vi "microspec_validating_v9.vi"() -> ()   [LabVIEW 2009]
uses:
  <vilib>/Utility/file.llb/Write To Spreadsheet File (string).vi
  <vilib>/Instr/_visa.llb/VISA Configure Serial Port (Instr).vi
panel:
  in  "Path":path
  in  "intergration time":dbl caption="sensor\nintergration time (us)" min=54.0 max=5000000.0 step=100.0
  in  "?":T1(tab)
  out "radiometer data file path":path
  in  "Runname":string
  out "Sensor_name":string
  out "Radiometer Average":dbl
  in  "Delay":dbl
  in  "Step":dbl
  in  "Stop Wl":dbl min=0.0 max=5000.0 step=100.0
  in  "Start Wl":dbl min=0.0 max=5000.0 step=100.0
  in  "mean_number":i32 caption="Mean Number"
  out "Current Wavelength":dbl
  out "XY-Graph 2":cluster{"Y":dbl[], "Y":dbl[]}[](graph)
  in  "run 5":bool
  out "sectrometer data file path":path
  in  "save data":bool
  in  "reset with every wavelength?":bool caption="reset with new run?"
  in  "Delay":dbl
  in  "Step":dbl
  in  "Stop Wl":dbl min=0.0 max=5000.0 step=100.0
  out "Current Wavelength":dbl
  in  "Start Wl 2":dbl min=0.0 max=5000.0 step=10.0
  in  "Sensor":string(combo)
  in  "run 2":bool
  in  "Set Runs":i32
  out "Current Run":i32
  in  "stop runs":bool
  out "raw_data":cluster{"Y":dbl[], "Y":dbl[]}[](graph) caption="raw data"
  out "raw_data 2":cluster{"Y":dbl[], "Y":dbl[]}[](graph) caption="raw data"
  in  "Stopp":bool
  out "System Setup":i32
  out "DLL Version":string
  out "Get Version":i32
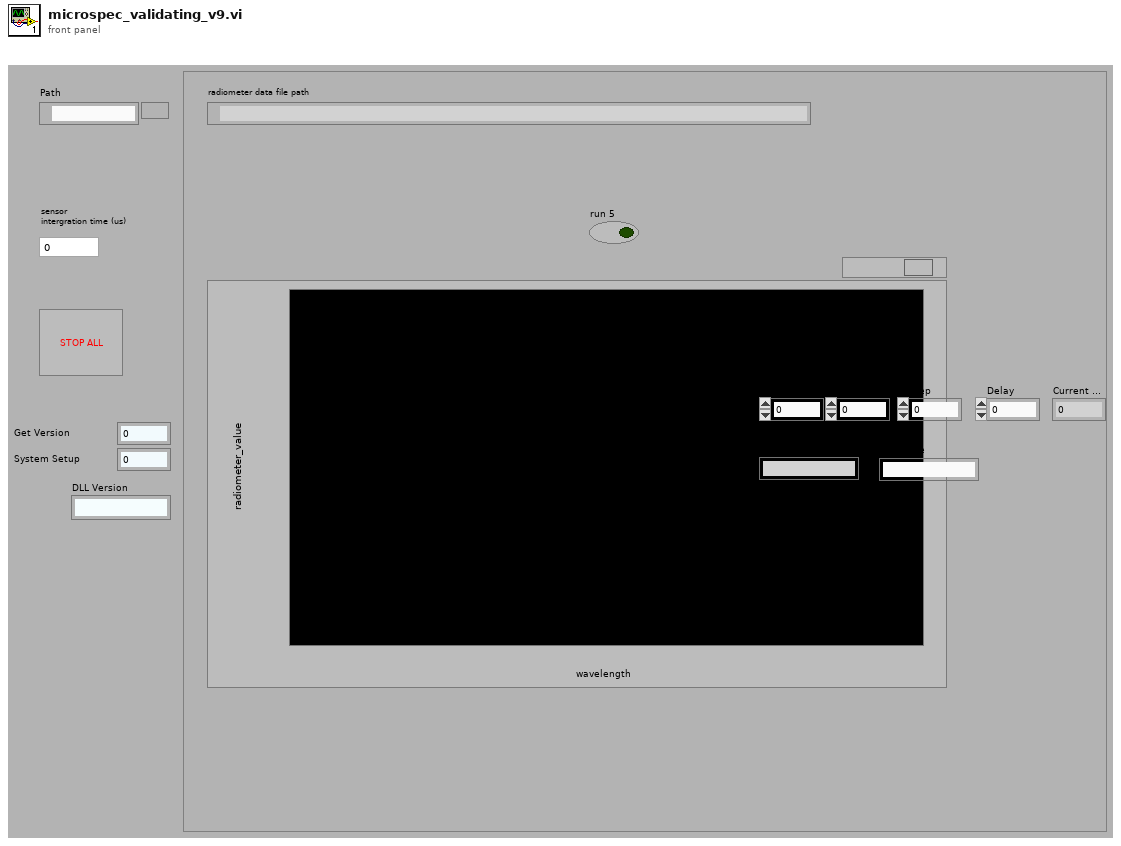
[diagram p1: front panel]
types:
  T1 = enum32{"radiometer calibration", "measuring sequence", "microspec standalone"}
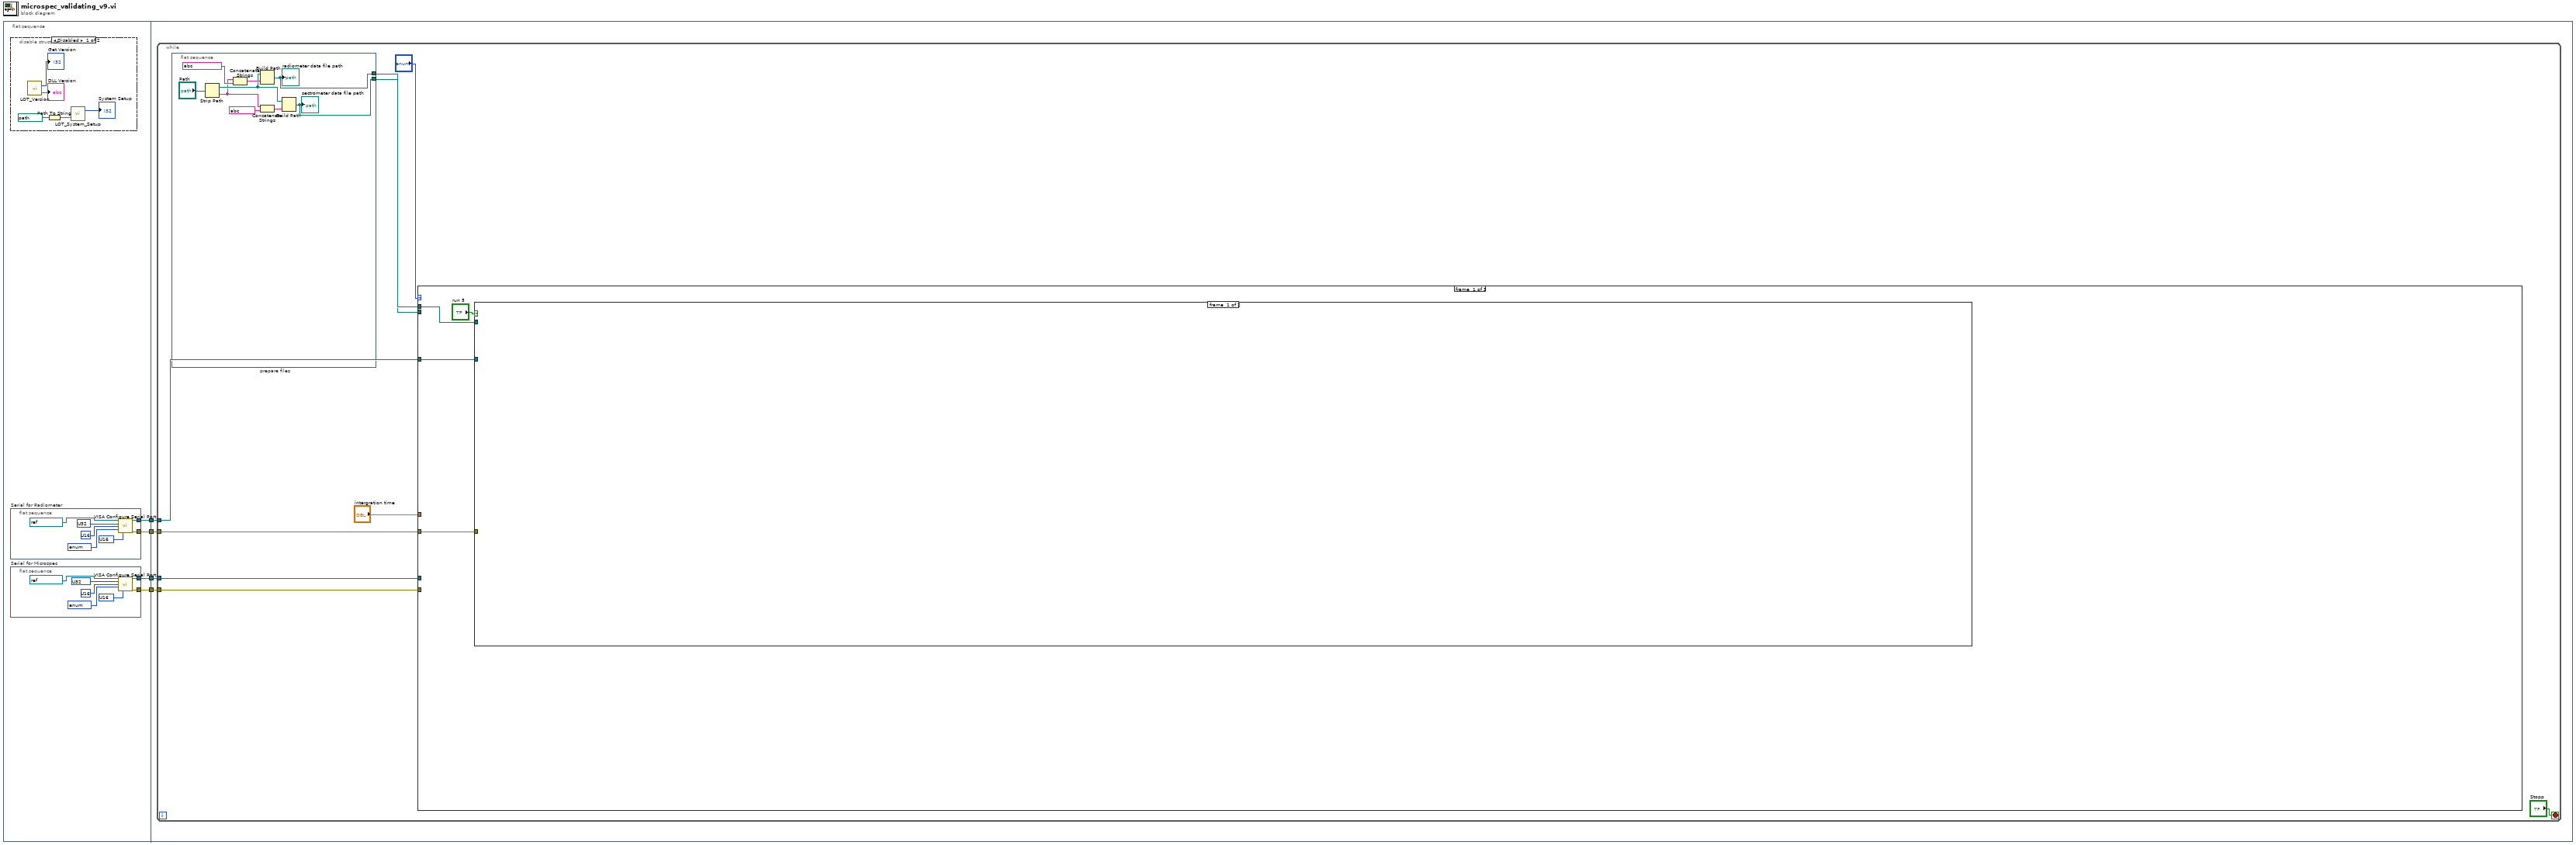
[diagram p0: block diagram]
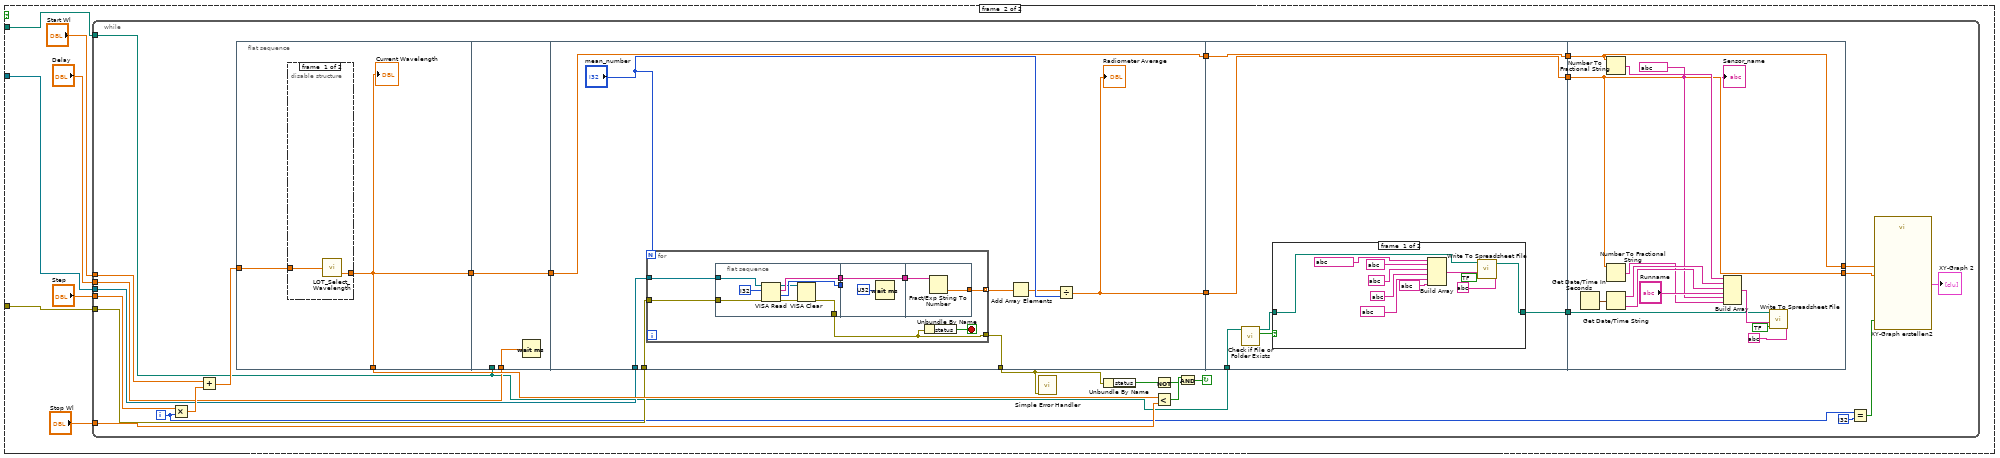
[diagram p3: hidden frame]
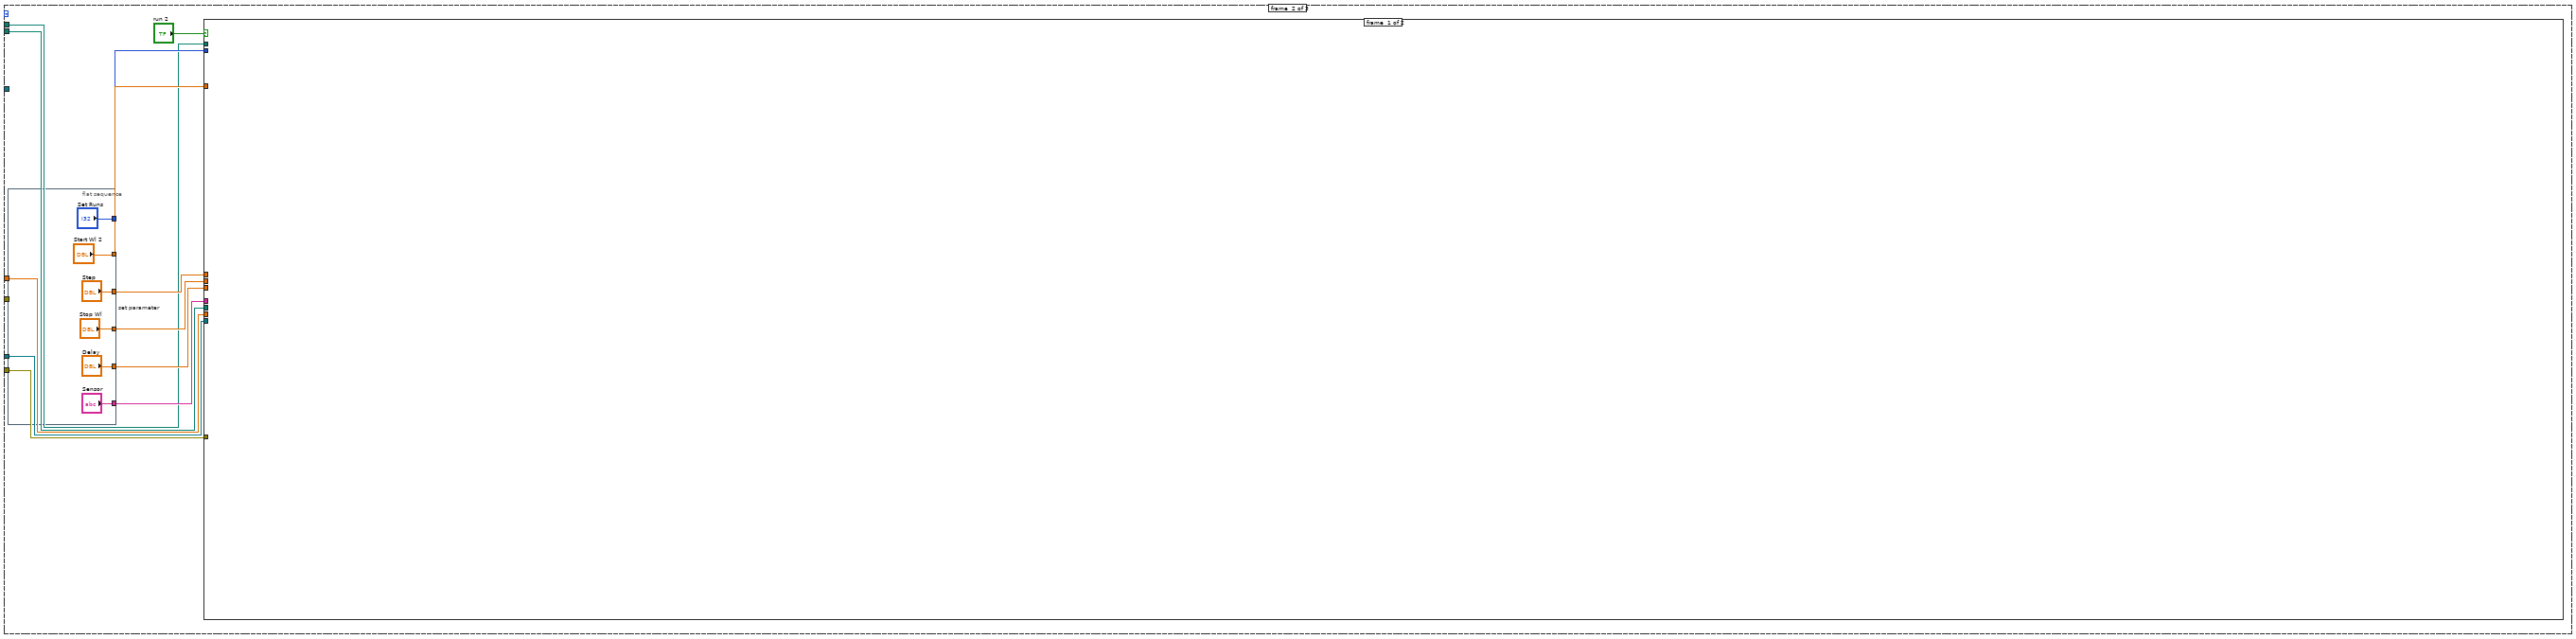
[diagram p6: hidden frame]
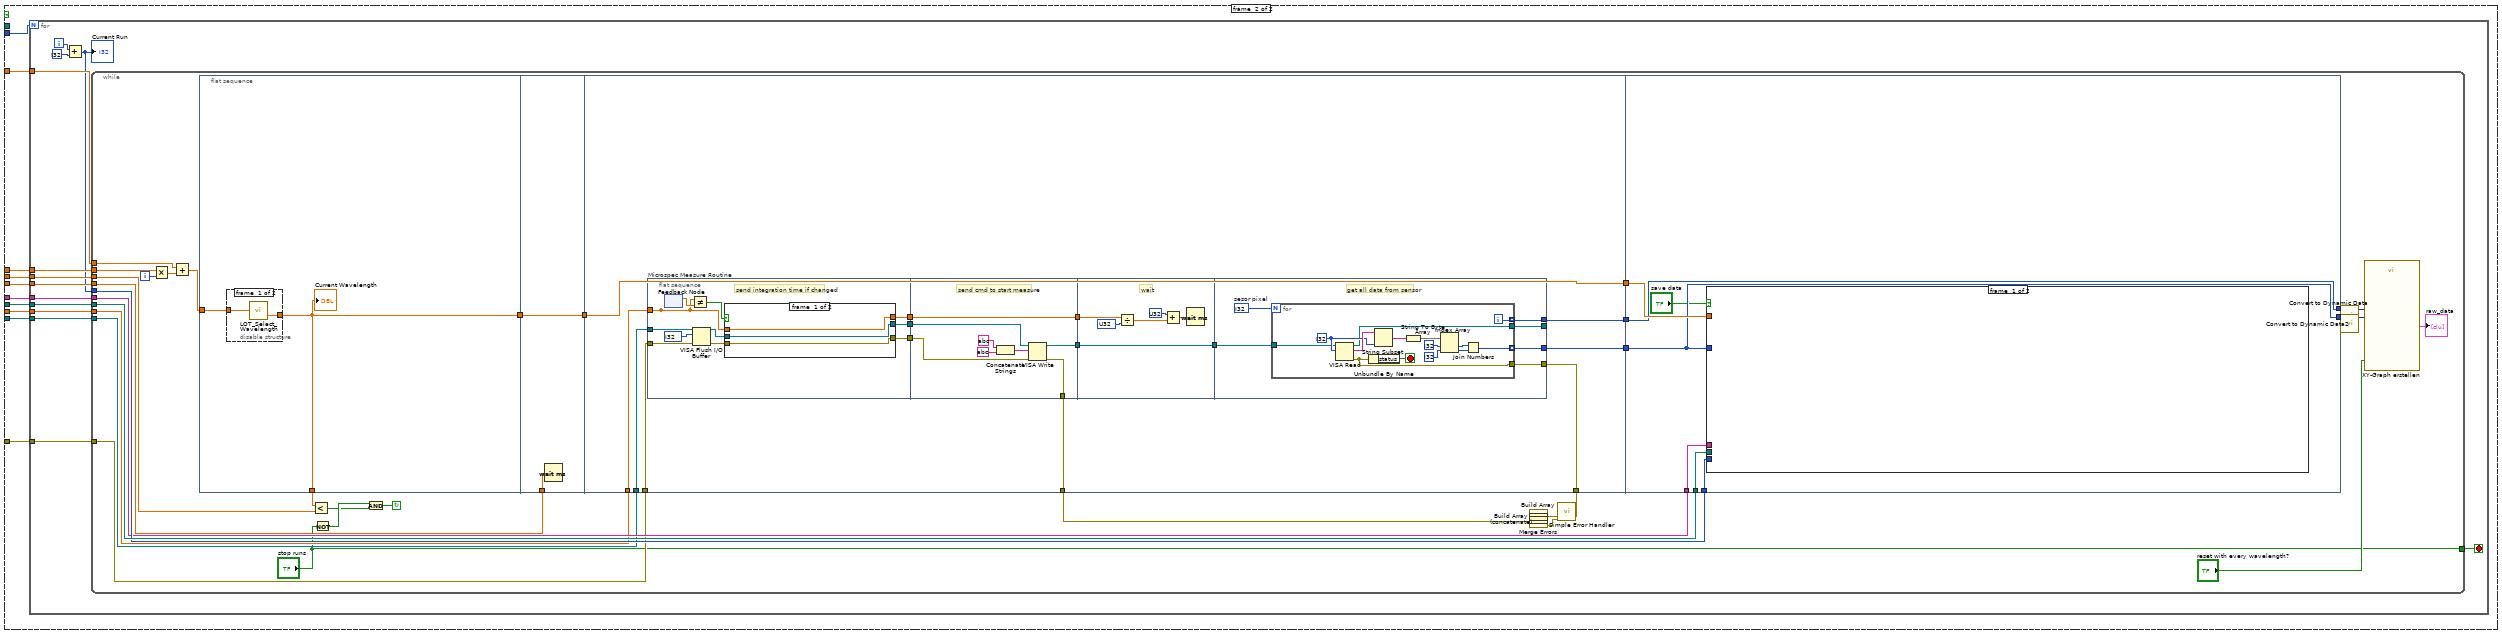
[diagram p7: hidden frame]
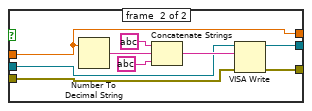
[diagram p9: hidden frame]
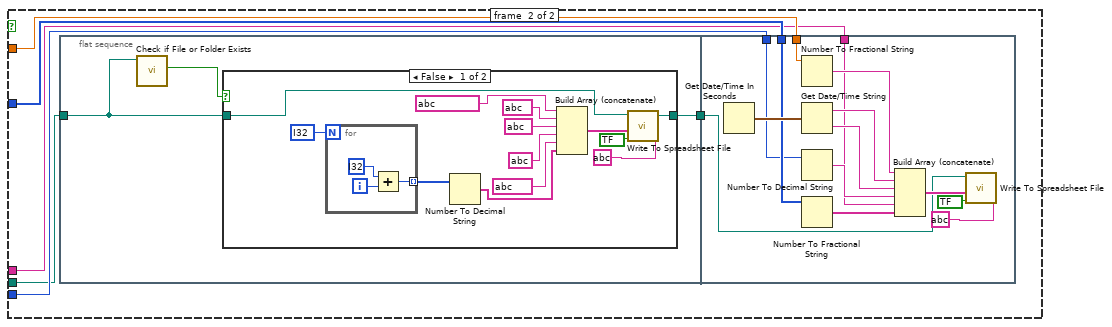
[diagram p10: hidden frame]
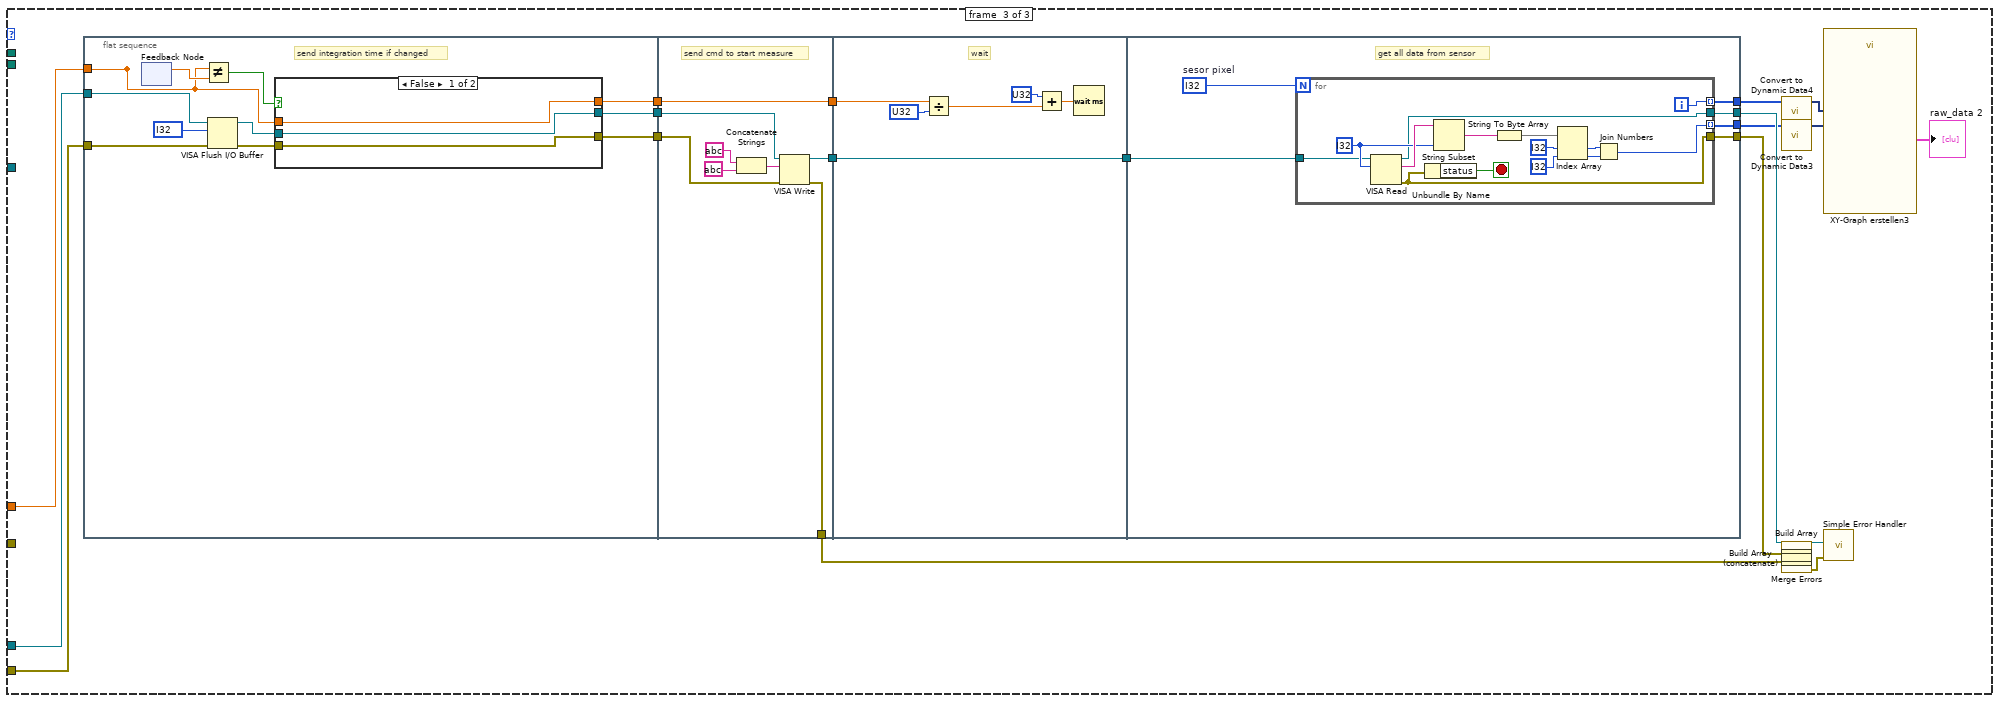
[diagram p12: hidden frame]
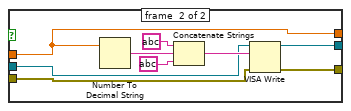
[diagram p13: hidden frame]
diagram:
  n1 = flat-sequence {
    tunnel: [w8] -> w4
    tunnel: [w7] -> w3
    tunnel: [w6] -> w2
    tunnel: [w5] -> w1
    tunnel: w4 -> [w31]
    tunnel: w3 -> [w30]
    tunnel: w2 -> [w29]
    tunnel: w1 -> [w28]
    frame #0 {
      # "Configuration"
      n2 = disable-structure shown="Disabled" {
        frame #0 {
          n3 = call "LOT_Version.vi"() -> ("Version"=→"DLL Version":string, "Get Version"=→"Get Version":i32)
          n4 = Path To String(path=path ? ("Configuration File")) -> (string=w25:string)
          n5 = call "LOT_System_Setup.vi"("CFG File Path"=w25) -> ("Error Code"=→"System Setup":i32)  [unwired: 2 in]
        }
        frame #1 {
        }
      }
      n6 = flat-sequence "Serial for Radiometer" {
        tunnel: [w15] -> w6
        tunnel: [w14] -> w5
        frame #0 {
          w10 = u16 ? items=["1.0", "1.5", "2.0"] ("stop bits (10: 1 bit)")
          n7 = call-poly "VISA Configure Serial Port"("VISA resource name"=refnum<visa-resource-name> ?, "baud rate (9600)"=u32 ?, "data bits (8)"=u16 ?, "parity (0:none)"=enum16{"None", "Odd", "Even", "Mark", "Space"} ?, "stop bits (10: 1 bit)"=w10) -> ("VISA resource name out"=w14:refnum<visa-resource-name>, "error out"=w15:errorcluster)  [unwired: 9 in]
        }
      }
      n8 = flat-sequence "Serial for Microspec" {
        tunnel: [w22] -> w8
        tunnel: [w21] -> w7
        frame #0 {
          w17 = u16 ? items=["1.0", "1.5", "2.0"] ("stop bits (10: 1 bit)")
          n9 = call-poly "VISA Configure Serial Port"("VISA resource name"=refnum<visa-resource-name> ?, "baud rate (9600)"=u32 ?, "data bits (8)"=u16 ?, "parity (0:none)"=enum16{"None", "Odd", "Even", "Mark", "Space"} ?, "stop bits (10: 1 bit)"=w17) -> ("VISA resource name out"=w22:refnum<visa-resource-name>, "error out"=w21:errorcluster)  [unwired: 9 in]
        }
      }
    }
    frame #1 {
      n10 = while {
        tunnel: w31 -> [w38]
        tunnel: w30 -> [w37]
        tunnel: w29 -> [w36]
        tunnel: w28 -> [w35]
        stop <- "Stopp" stop-if-true
        n11 = flat-sequence "prepare files" {
          tunnel: [w41] -> w32
          tunnel: [w42] -> w33
          frame #0 {
            n12 = Strip Path(path="Path") -> (stripped path=w44:path, name=w43:string)
            n13 = Concatenate Strings(w43, string ?) -> (w45:string)
            n14 = Build Path(base path=w44, name or relative path=w45) -> (appended path=w42:path)
            "radiometer data file path" <- w42
            n15 = Concatenate Strings(w43, string ?) -> (w47:string)
            n16 = Build Path(base path=w44, name or relative path=w47) -> (appended path=w41:path)
            "sectrometer data file path" <- w41
          }
        }
        n17 = case shown="\"measuring sequence\"" "?" {
          tunnel: w32 -> [_ w165 _]
          tunnel: w38 -> [_ w164 w374]
          tunnel: w37 -> [_ w163 w373]
          tunnel: w36 -> [w52 _ _]
          tunnel: w35 -> [w51 _ _]
          tunnel: "intergration time" -> [_ w162 w372]
          tunnel: w33 -> [w50 w155 _]
          frame #0 {
            n18 = case shown="True" "run 5" {
              tunnel: w50 -> [_ w56]
              tunnel: w52 -> [_ w55]
              tunnel: w51 -> [_ w54]
              frame #0 {
              }
              frame #1 {
                n19 = while {
                  tunnel: "Step" -> [w88]
                  tunnel: "Start Wl" -> [w86]
                  tunnel: "Stop Wl" -> [w85]
                  tunnel: "Delay" -> [w81]
                  tunnel: w56 -> [w67]
                  tunnel: w54 -> [w80]
                  tunnel: w55 -> [w79]
                  i -> [w75]
                  stop <- w62 continue-if-true
                  n20 = Multiply(x=w88, y=w75) -> (x*y=w87:dbl)
                  n21 = Add(x=w86, y=w87) -> (x+y=w84:dbl)
                  n22 = flat-sequence {
                    tunnel: w84 -> [w90]
                    tunnel: [w89] -> w83
                    tunnel: [w89] -> w82
                    tunnel: w67 -> [_]
                    tunnel: w82 -> [w94]
                    tunnel: w81 -> [w95]
                    tunnel: [w94] -> w78
                    tunnel: w80 -> [w103]
                    tunnel: w79 -> [w102]
                    tunnel: w78 -> [w101]
                    tunnel: [w101] -> w71
                    tunnel: [w99] -> w69
                    tunnel: [w96] -> w61
                    tunnel: w71 -> [w129]
                    tunnel: [w129] -> w70
                    tunnel: w69 -> [w128]
                    tunnel: [w128] -> w68
                    tunnel: w67 -> [w126]
                    tunnel: [w127] -> w66
                    tunnel: [w145] -> w72
                    tunnel: [w146] -> w76
                    tunnel: w70 -> [w146]
                    tunnel: w68 -> [w145]
                    tunnel: w66 -> [w148]
                    frame #0 {
                      n23 = disable-structure shown="Enabled" {
                        disable-tunnel: w90 -> [w92 w93]
                        disable-tunnel: [w91 w93] -> w89
                        frame #0 {
                          n24 = call "LOT_Select_Wavelength.vi"("Input Wavelength"=w92) -> ("Current Wavelength"=w91:dbl)  [unwired: 1 out]
                        }
                        frame #1 {
                        }
                      }
                      "Current Wavelength" <- w89
                    }
                    frame #1 {
                      n25 = Wait (ms)(milliseconds to wait=w95) -> ()  [unwired: 1 out]
                    }
                    frame #2 {
                      n26 = for {
                        N: "mean_number" -> [_]
                        tunnel: w103 -> [w108]
                        tunnel: w102 -> [w107]
                        tunnel: [w106] -> w97 mode=indexing
                        tunnel: [w105] -> w96
                        stop <- w104 stop-if-true
                        n27 = flat-sequence {
                          tunnel: [w116] -> w111
                          tunnel: w108 -> [w119]
                          tunnel: w107 -> [w118]
                          tunnel: [w115] -> w110
                          tunnel: [w112] -> w105
                          tunnel: w111 -> [w121]
                          tunnel: [w121] -> w109
                          tunnel: w110 -> [_]
                          tunnel: w109 -> [w122]
                          tunnel: [w123] -> w106
                          frame #0 {
                            n28 = VISA Read(VISA resource name=w119, byte count=i32 ?, error in (no error)=w118) -> (VISA resource name out=w113:refnum<visa-resource-name>, read buffer=w116:string, return count=w115:u32, error out=w114:errorcluster)
                            n29 = VISA Clear(VISA resource name=w113, error in (no error)=w114) -> (error out=w112:errorcluster)  [unwired: 1 out]
                          }
                          frame #1 {
                            n30 = Wait (ms)(milliseconds to wait=u32 ? ("Zu wartende ms")) -> ()  [unwired: 1 out]
                          }
                          frame #2 {
                            n31 = Fract/Exp String To Number(string=w122) -> (number=w123:dbl)  [unwired: 3 in, 1 out]
                          }
                        }
                        n32 = Unbundle By Name(w105) -> ("status"=w104:bool)
                      }
                      n33 = Add Array Elements(numeric array=w97) -> (sum=w98:dbl)
                      n34 = Divide(x=w98, y="mean_number") -> (x/y=w99:dbl)
                      "Radiometer Average" <- w99
                    }
                    frame #3 {
                      n35 = call <vilib>:"Check if File or Folder Exists.vi"("path"=w126) -> ("file or folder exists?"=w125:bool, "dup path"=w124:path)  [unwired: 8 in, 1 out]
                      n36 = case shown="True" w125 {
                        tunnel: w124 -> [w138 w141]
                        tunnel: [w131 w141] -> w127
                        frame #0 {
                          n37 = Build Array(string ?, string ? ("Element"), string ? ("Element"), string ? ("Element"), string ? ("Element"), string ?) -> (w140:string[])
                          n38 = call-poly <vilib>:"Write To Spreadsheet File.vi"("delimiter (\\t)"=string ?, "append to file? (new file:F)"=bool ?, "1D data"=w140, "file path (dialog if empty)"=w138) -> ("new file path (Not A Path if cancelled)"=w131:path)  [unwired: 4 in]
                        }
                        frame #1 {
                        }
                      }
                    }
                    frame #4 {
                      w143 = string ? ("Sensor_name")
                      n39 = Get Date/Time In Seconds() -> (seconds since 1Jan1904=w153:timestamp)
                      n40 = Number To Fractional String(number=w146) -> (F-format string=w154:string)  [unwired: 3 in]
                      n41 = Number To Fractional String(number=w145) -> (F-format string=w142:string)  [unwired: 3 in]
                      n42 = Get Date/Time String(seconds (now)=w153) -> (date string=w152:string, time string=w151:string)  [unwired: 2 in]
                      n43 = Build Array(w154, w152, w151, "Runname", w143, w142) -> (w150:string[])
                      n44 = call-poly <vilib>:"Write To Spreadsheet File.vi"("delimiter (\\t)"=string ?, "append to file? (new file:F)"=bool ?, "1D data"=w150, "file path (dialog if empty)"=w148) -> ()  [unwired: 4 in, 1 out]
                      "Sensor_name" <- w143
                    }
                  }
                  n45 = call <vilib>:"Simple Error Handler.vi"("error in (no error)"=w61) -> ()  [unwired: 4 in, 5 out]
                  n46 = Unbundle By Name(w61) -> ("status"=w63:bool)
                  n47 = Less?(x=w83, y=w85) -> (x < y?=w65:bool)
                  n48 = Not(x=w63) -> (.not. x?=w64:bool)
                  n49 = And(x=w65, y=w64) -> (x .and. y?=w62:bool)
                  n50 = Equal?(x=w75, y=i32 ?) -> (x = y?=w73:bool)
                  n51 = call "XY-Graph erstellen2"("Reset"=w73, "Y Input"=w72, "X Input"=w76) -> ("XY Graph"=→"XY-Graph 2":cluster{"Y":dbl[], "Y":dbl[]}[])  [unwired: 7 in, 1 out]
                }
              }
            }
          }
          frame #1 {
            n52 = flat-sequence "set parameter" {
              tunnel: ["Sensor"] -> w161
              tunnel: ["Delay"] -> w160
              tunnel: ["Step"] -> w159
              tunnel: ["Stop Wl"] -> w158
              tunnel: ["Start Wl 2"] -> w157
              tunnel: ["Set Runs"] -> w156
              frame #0 {
              }
            }
            n53 = case shown="True" "run 2" {
              tunnel: w165 -> [_ w173]
              tunnel: w161 -> [_ w182]
              tunnel: w156 -> [_ w181]
              tunnel: w164 -> [_ w180]
              tunnel: w163 -> [_ w179]
              tunnel: w160 -> [_ w178]
              tunnel: w158 -> [_ w177]
              tunnel: w159 -> [_ w176]
              tunnel: w157 -> [_ w175]
              tunnel: w162 -> [_ w174]
              tunnel: w155 -> [_ _]
              frame #0 {
              }
              frame #1 {
                n54 = for {
                  N: w181 -> [_]
                  tunnel: w173 -> [w195]
                  tunnel: w182 -> [w194]
                  tunnel: w180 -> [w193]
                  tunnel: w179 -> [w192]
                  tunnel: w178 -> [w191]
                  tunnel: w177 -> [w190]
                  tunnel: w176 -> [w189]
                  tunnel: w175 -> [w188]
                  tunnel: w174 -> [w187]
                  i -> [w186]
                  stop <- w183 stop-if-true
                  n55 = Add(x=w186, y=i32 ?) -> (x+y=w185:i32)
                  "Current Run" <- w185
                  n56 = while {
                    tunnel: w195 -> [w227]
                    tunnel: w185 -> [w226]
                    tunnel: w194 -> [w222]
                    tunnel: w193 -> [w220]
                    tunnel: w192 -> [w219]
                    tunnel: w191 -> [w210]
                    tunnel: w190 -> [w208]
                    tunnel: w189 -> [w207]
                    tunnel: w188 -> [w206]
                    tunnel: w187 -> [w205]
                    tunnel: ["stop runs"] -> w183
                    i -> [w224]
                    stop <- w199 continue-if-true
                    n57 = Multiply(x=w207, y=w224) -> (x*y=w229:dbl)
                    n58 = Add(x=w206, y=w229) -> (x+y=w228:dbl)
                    n59 = flat-sequence {
                      tunnel: w228 -> [w231]
                      tunnel: [w230] -> w225
                      tunnel: [w230] -> w209
                      tunnel: w225 -> [w235]
                      tunnel: w210 -> [w236]
                      tunnel: [w235] -> w213
                      tunnel: [w239] -> w221
                      tunnel: w220 -> [w243]
                      tunnel: w219 -> [w244]
                      tunnel: [w242] -> w217
                      tunnel: [w241] -> w216
                      tunnel: [w240] -> w215
                      tunnel: w213 -> [w239]
                      tunnel: w205 -> [w238]
                      tunnel: [w237] -> w204
                      tunnel: w227 -> [w314]
                      tunnel: w221 -> [w313]
                      tunnel: w226 -> [w312]
                      tunnel: [w310] -> w211
                      tunnel: w222 -> [w311]
                      tunnel: w215 -> [w310]
                      tunnel: w204 -> [w309]
                      tunnel: [w309] -> w203
                      frame #0 {
                        # "set wavelength"
                        n60 = disable-structure shown="Enabled" {
                          disable-tunnel: w231 -> [w233 w234]
                          disable-tunnel: [w232 w234] -> w230
                          frame #0 {
                            n61 = call "LOT_Select_Wavelength.vi"("Input Wavelength"=w233) -> ("Current Wavelength"=w232:dbl)  [unwired: 1 out]
                          }
                          frame #1 {
                          }
                        }
                        "Current Wavelength" <- w230
                      }
                      frame #1 {
                        # "wait"
                        n62 = Wait (ms)(milliseconds to wait=w236) -> ()  [unwired: 1 out]
                      }
                      frame #2 {
                        n63 = flat-sequence "Microspec Measure Routine" {
                          tunnel: w243 -> [w252]
                          tunnel: w244 -> [w261]
                          tunnel: [w256] -> w250
                          tunnel: [w255] -> w249
                          tunnel: [w254] -> w248
                          tunnel: w238 -> [w251]
                          tunnel: [w278] -> w247
                          tunnel: [w277] -> w241
                          tunnel: w250 -> [w275]
                          tunnel: w249 -> [w276]
                          tunnel: w248 -> [w274]
                          tunnel: [w274] -> w246
                          tunnel: w247 -> [w283]
                          tunnel: [w283] -> w245
                          tunnel: w246 -> [w282]
                          tunnel: w245 -> [w293]
                          tunnel: [w292] -> w240
                          tunnel: [w291] -> w237
                          tunnel: [w289] -> _
                          tunnel: [w288] -> w242
                          frame #0 {
                            # "send integration time if changed"
                            n64 = feedback #1() -> (w260:dbl)  [unwired: 1 in]
                            n65 = Not Equal?(x=w251, y=w260) -> (x != y?=w259:bool)
                            n66 = VISA Flush I/O Buffer(VISA resource name=w252, mask (16)=i32 ?, error in (no error)=w261) -> (VISA resource name out=w258:refnum<visa-resource-name>, error out=w257:errorcluster)
                            n67 = case shown="True" w259 {
                              tunnel: w258 -> [w263 w269]
                              tunnel: w257 -> [w262 w268]
                              tunnel: [w262 w267] -> w256
                              tunnel: [w263 w266] -> w255
                              tunnel: w251 -> [w264 w265]
                              tunnel: [w264 w265] -> w254
                              frame #0 {
                              }
                              frame #1 {
                                n68 = Number To Decimal String(number=w265) -> (decimal integer string=w272:string)  [unwired: 1 in]
                                n69 = Concatenate Strings(string ?, w272, string ?) -> (w270:string)
                                n70 = VISA Write(VISA resource name=w269, write buffer=w270, error in (no error)=w268) -> (VISA resource name out=w266:refnum<visa-resource-name>, error out=w267:errorcluster)  [unwired: 1 out]
                              }
                            }
                          }
                          frame #1 {
                            # "send cmd to start measure"
                            n71 = Concatenate Strings(string ?, string ?) -> (w279:string)
                            n72 = VISA Write(VISA resource name=w276, write buffer=w279, error in (no error)=w275) -> (VISA resource name out=w278:refnum<visa-resource-name>, error out=w277:errorcluster)  [unwired: 1 out]
                          }
                          frame #2 {
                            # "wait"
                            n73 = Divide(x=w282, y=u32 ? ("Zu wartende ms")) -> (x/y=w284:dbl)
                            n74 = Add(x=u32 ? ("Zu wartende ms"), y=w284) -> (x+y=w286:dbl)
                            n75 = Wait (ms)(milliseconds to wait=w286) -> ()  [unwired: 1 out]
                          }
                          frame #3 {
                            w290 = i32 ?  # sesor pixel
                            # "get all data from sensor"
                            n76 = for {
                              N: w290 -> [_]
                              tunnel: w293 -> [w297]
                              tunnel: [w299] -> w292 mode=indexing
                              tunnel: [w298] -> w291 mode=indexing
                              tunnel: [w295] -> w289
                              tunnel: [w294] -> w288
                              i -> [w298]
                              stop <- w296 stop-if-true
                              w306 = i32 ?
                              n77 = VISA Read(VISA resource name=w297, byte count=w306) -> (VISA resource name out=w295:refnum<visa-resource-name>, read buffer=w307:string, error out=w294:errorcluster)  [unwired: 1 in, 1 out]
                              n78 = Unbundle By Name(w294) -> ("status"=w296:bool)
                              n79 = String Subset(string=w307, length (rest)=w306) -> (substring=w305:string)  [unwired: 1 in]
                              n80 = String To Byte Array(string=w305) -> (unsigned byte array=w304:u8[])
                              n81 = Index Array(array=w304, index #1=i32 ?, index #2=i32 ?) -> (element #1=w300:u8, element #2=w301:u8)
                              n82 = Join Numbers(hi=w300, lo=w301) -> ((hi.lo)=w299:u16)
                            }
                          }
                        }
                      }
                      frame #3 {
                        n83 = case shown="True" "save data" {
                          tunnel: w314 -> [_ w317]
                          tunnel: w313 -> [_ w319]
                          tunnel: w312 -> [_ w318]
                          tunnel: w310 -> [_ w320]
                          tunnel: w311 -> [_ w316]
                          frame #0 {
                          }
                          frame #1 {
                            n84 = flat-sequence {
                              tunnel: w317 -> [w323]
                              tunnel: [w321] -> w315
                              tunnel: w320 -> [w347]
                              tunnel: w319 -> [w346]
                              tunnel: w318 -> [w345]
                              tunnel: w316 -> [w343]
                              tunnel: w315 -> [w341]
                              frame #0 {
                                n85 = call <vilib>:"Check if File or Folder Exists.vi"("path"=w323) -> ("file or folder exists?"=w322:bool)  [unwired: 8 in, 2 out]
                                n86 = case shown="False" w322 {
                                tunnel: w323 -> [w327 w340]
                                tunnel: [w324 w340] -> w321
                                frame #0 {
                                n87 = for {
                                N: i32 ? -> [_]
                                tunnel: [w337] -> w330 mode=indexing
                                i -> [w339]
                                n88 = Add(x=i32 ?, y=w339) -> (x+y=w337:i32)
                                }
                                n89 = Number To Decimal String(number=w330) -> (decimal integer string=w332:string[])  [unwired: 1 in]
                                n90 = Build Array (concatenate)(string ?, string ? ("Element"), string ? ("Element"), string ? ("Element"), string ? ("Element"), w332) -> (w336:string[])
                                n91 = call-poly <vilib>:"Write To Spreadsheet File.vi"("delimiter (\\t)"=string ?, "append to file? (new file:F)"=bool ?, "1D data"=w336, "file path (dialog if empty)"=w327) -> ("new file path (Not A Path if cancelled)"=w324:path)  [unwired: 4 in]
                                }
                                frame #1 {
                                }
                                }
                              }
                              frame #1 {
                                n92 = Get Date/Time In Seconds() -> (seconds since 1Jan1904=w349:timestamp)
                                n93 = Number To Fractional String(number=w346) -> (F-format string=w348:string)  [unwired: 3 in]
                                n94 = Get Date/Time String(seconds (now)=w349) -> (date string=w350:string, time string=w351:string)  [unwired: 2 in]
                                n95 = Number To Decimal String(number=w345) -> (decimal integer string=w344:string)  [unwired: 1 in]
                                n96 = Number To Fractional String(number=w347) -> (F-format string=w354:string[])  [unwired: 3 in]
                                n97 = Build Array (concatenate)(w348, w350, w351, w344, w343, w354) -> (w352:string[])
                                n98 = call-poly <vilib>:"Write To Spreadsheet File.vi"("delimiter (\\t)"=string ?, "append to file? (new file:F)"=bool ?, "1D data"=w352, "file path (dialog if empty)"=w341) -> ()  [unwired: 4 in, 1 out]
                              }
                            }
                          }
                        }
                      }
                    }
                    n99 = Less?(x=w209, y=w208) -> (x < y?=w200:bool)
                    n100 = Not(x="stop runs") -> (.not. x?=w201:bool)
                    n101 = And(x=w201, y=w200) -> (x .and. y?=w199:bool)
                    n102 = Build Array(w217, w216) -> (w197:errorcluster[])
                    n103 = Build Array (concatenate)(w197) -> (w196:errorcluster[])
                    n104 = call <vilib>:"Merge Errors.vi"("error array in"=w196) -> ("error out"=w218:errorcluster)  [unwired: 6 in]
                    n105 = call <vilib>:"Simple Error Handler.vi"("error in (no error)"=w218) -> ()  [unwired: 4 in, 5 out]
                    n106 = call "Convert to Dynamic Data"("Array"=w203) -> ("Dynamic Data Type"=w212:dynamicdata)  [unwired: 3 in]
                    n107 = call "Convert to Dynamic Data2"("Array"=w211) -> ("Dynamic Data Type"=w214:dynamicdata)  [unwired: 3 in]
                    n108 = call "XY-Graph erstellen"("Reset"="reset with every wavelength?", "Y Input"=w214, "X Input"=w212) -> ("XY Graph"=→"raw_data":cluster{"Y":dbl[], "Y":dbl[]}[])  [unwired: 7 in, 1 out]
                  }
                }
              }
            }
          }
          frame #2 {
            n109 = flat-sequence {
              tunnel: w374 -> [w384]
              tunnel: w373 -> [w385]
              tunnel: [w379] -> w371
              tunnel: [w378] -> w370
              tunnel: [w377] -> w369
              tunnel: w372 -> [w375]
              tunnel: [w402] -> w368
              tunnel: [w401] -> w364
              tunnel: w371 -> [w399]
              tunnel: w370 -> [w400]
              tunnel: w369 -> [w398]
              tunnel: [w398] -> w367
              tunnel: w368 -> [w407]
              tunnel: [w407] -> w366
              tunnel: w367 -> [w406]
              tunnel: w366 -> [w416]
              tunnel: [w417] -> w365
              tunnel: [w415] -> w358
              tunnel: [w414] -> w357
              tunnel: [w412] -> w362
              frame #0 {
                # "send integration time if changed"
                n110 = feedback #2() -> (w383:dbl)  [unwired: 1 in]
                n111 = Not Equal?(x=w375, y=w383) -> (x != y?=w382:bool)
                n112 = VISA Flush I/O Buffer(VISA resource name=w384, mask (16)=i32 ?, error in (no error)=w385) -> (VISA resource name out=w381:refnum<visa-resource-name>, error out=w380:errorcluster)
                n113 = case shown="False" w382 {
                  tunnel: w381 -> [w387 w393]
                  tunnel: w380 -> [w386 w392]
                  tunnel: [w386 w391] -> w379
                  tunnel: [w387 w390] -> w378
                  tunnel: w375 -> [w388 w389]
                  tunnel: [w388 w389] -> w377
                  frame #0 {
                  }
                  frame #1 {
                    n114 = Number To Decimal String(number=w389) -> (decimal integer string=w396:string)  [unwired: 1 in]
                    n115 = Concatenate Strings(string ?, w396, string ?) -> (w394:string)
                    n116 = VISA Write(VISA resource name=w393, write buffer=w394, error in (no error)=w392) -> (VISA resource name out=w390:refnum<visa-resource-name>, error out=w391:errorcluster)  [unwired: 1 out]
                  }
                }
              }
              frame #1 {
                # "send cmd to start measure"
                n117 = Concatenate Strings(string ?, string ?) -> (w403:string)
                n118 = VISA Write(VISA resource name=w400, write buffer=w403, error in (no error)=w399) -> (VISA resource name out=w402:refnum<visa-resource-name>, error out=w401:errorcluster)  [unwired: 1 out]
              }
              frame #2 {
                # "wait"
                n119 = Divide(x=w406, y=u32 ? ("Zu wartende ms")) -> (x/y=w408:dbl)
                n120 = Add(x=u32 ? ("Zu wartende ms"), y=w408) -> (x+y=w410:dbl)
                n121 = Wait (ms)(milliseconds to wait=w410) -> ()  [unwired: 1 out]
              }
              frame #3 {
                w413 = i32 ?  # sesor pixel
                # "get all data from sensor"
                n122 = for {
                  N: w413 -> [_]
                  tunnel: w416 -> [w421]
                  tunnel: [w420] -> w417
                  tunnel: [w423] -> w415 mode=indexing
                  tunnel: [w422] -> w414 mode=indexing
                  tunnel: [w418] -> w412
                  i -> [w422]
                  stop <- w419 stop-if-true
                  w430 = i32 ?
                  n123 = VISA Read(VISA resource name=w421, byte count=w430) -> (VISA resource name out=w418:refnum<visa-resource-name>, read buffer=w431:string, error out=w420:errorcluster)  [unwired: 1 in, 1 out]
                  n124 = Unbundle By Name(w420) -> ("status"=w419:bool)
                  n125 = String Subset(string=w431, length (rest)=w430) -> (substring=w429:string)  [unwired: 1 in]
                  n126 = String To Byte Array(string=w429) -> (unsigned byte array=w428:u8[])
                  n127 = Index Array(array=w428, index #1=i32 ?, index #2=i32 ?) -> (element #1=w424:u8, element #2=w425:u8)
                  n128 = Join Numbers(hi=w424, lo=w425) -> ((hi.lo)=w423:u16)
                }
              }
            }
            n129 = call "Convert to Dynamic Data4"("Array"=w357) -> ("Dynamic Data Type"=w359:dynamicdata)  [unwired: 3 in]
            n130 = call "Convert to Dynamic Data3"("Array"=w358) -> ("Dynamic Data Type"=w360:dynamicdata)  [unwired: 3 in]
            n131 = Build Array(w365, w364) -> (w356:errorcluster[])
            n132 = Build Array (concatenate)(w356) -> (w355:errorcluster[])
            n133 = call <vilib>:"Merge Errors.vi"("error array in"=w355) -> ("error out"=w363:errorcluster)  [unwired: 6 in]
            n134 = call "XY-Graph erstellen3"("Y Input"=w360, "X Input"=w359) -> ("XY Graph"=→"raw_data 2":cluster{"Y":dbl[], "Y":dbl[]}[])  [unwired: 8 in, 1 out]
            n135 = call <vilib>:"Simple Error Handler.vi"("error source (\" \")"=w362, "error in (no error)"=w363) -> ()  [unwired: 3 in, 5 out]
          }
        }
      }
    }
  }
